vi "Async Start video from CamServer (for web monitoring).vi"(1 "Camera":T1="Travcam") -> (0 "Error out":errorcluster)   [LabVIEW 2015]
uses:
  Y:/Temporary for transfer/Video server tests/ctls/Camera enum.ctl
panel:
  # "PN 21/08/15"
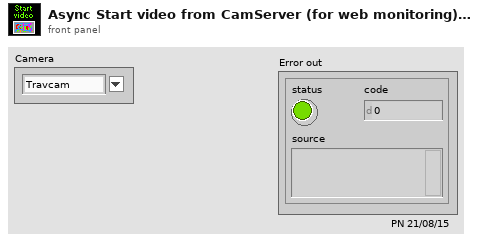
[diagram p1: front panel]
types:
  T1 = typedef "Camera enum.ctl" = string
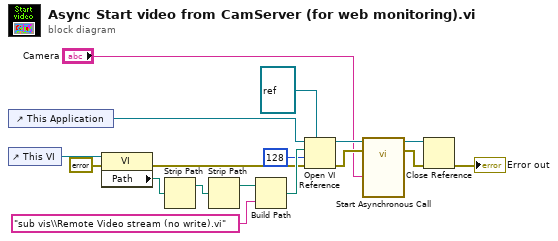
[diagram p0: block diagram]
diagram:
  n1 = control-ref of="This Application"() -> (w12:refnum<vi>)
  n2 = control-ref of="This VI"() -> (w17:refnum<vi>)
  n3 = property class="VI"(reference=w17, error in=errorcluster {"status"=FALSE, "code"=0, "source"=""} ("error in (no error)")) -> (error out=w14:errorcluster, "Path"=w10:path)  [unwired: 1 out]
  n4 = Strip Path(path=w10) -> (stripped path=w2:path)  [unwired: 1 out]
  n5 = Strip Path(path=w2) -> (stripped path=w1:path)  [unwired: 1 out]
  n6 = Build Path(base path=w1, name or relative path="sub vis\\Remote Video stream (no write).vi") -> (appended path=w15:path)
  n7 = Open VI Reference(type specifier VI Refnum (for type only)=refnum<vi> refnum, application reference (local)=w12, vi path=w15, options=128, error in (no error)=w14) -> (vi reference=w9:refnum<vi>, error out=w8:errorcluster)  [unwired: 1 in]
  n8 = call-by-ref "Start Asynchronous Call"(reference=w9, error in=w8, "Camera"="Camera") -> (reference out=w5:refnum<vi>, error out=w4:errorcluster)  [unwired: 1 out]
  n9 = Close Reference(reference=w5, error in (no error)=w4) -> (error out=→"Error out":errorcluster)
